vi "EpochConverter.vi"(11 "Epoch time":dbl format="%.7f") -> (0 "Date":string, 3 "String":string)   [LabVIEW 2015]
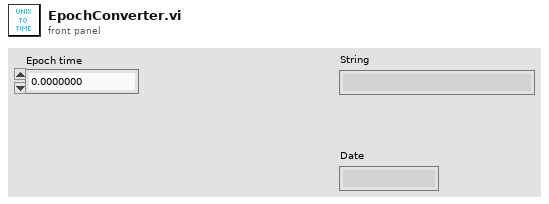
[diagram p1: front panel]
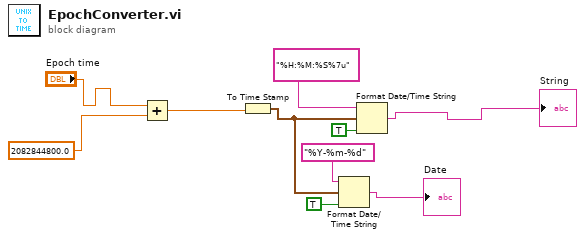
[diagram p0: block diagram]
diagram:
  n1 = Add(x="Epoch time", y=2082844800.0) -> (x+y=w9:dbl)
  n2 = To Time Stamp(1:w9) -> (0:w6:timestamp)
  n3 = Format Date/Time String(time format string (%c)="%Y-%m-%d", seconds (now)=w6, UTC format=TRUE) -> (date/time string=→"Date":string)
  n4 = Format Date/Time String(time format string (%c)="%H:%M:%S%7u", seconds (now)=w6, UTC format=TRUE) -> (date/time string=→"String":string)
